vi "Drive Arcade.vi"(8 "error in":errorcluster, 9 "Force? (F)":bool, 10 "Y Axis":dbl, 11 "X Axis":dbl) -> (0 "error out":errorcluster)   [LabVIEW 2016, in "Drive System.lvlib"]
uses:
  Drive System.lvlib
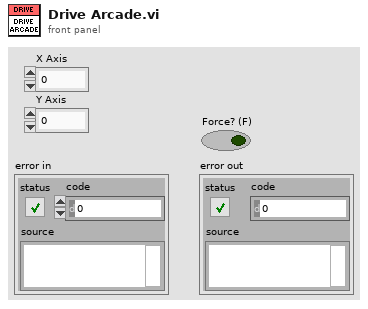
[diagram p1: front panel]
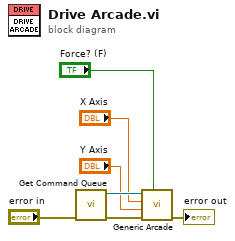
[diagram p0: block diagram]
diagram:
  n1 = call "Get Command Queue.vi"("error in (no error)"="error in") -> ("error out"=w5:errorcluster, "Queue out"=w4:refnum<queue>)  [unwired: 9 in]
  n2 = call "Generic Arcade.vi"("Force? (F)"="Force? (F)", "error in (no error)"=w5, "Y Axis"="Y Axis", "X Axis"="X Axis", "Queue in"=w4) -> ("error out"=→"error out":errorcluster)  [unwired: 6 in]
